vi "RP convert sweep.vi"(6 "Compact":bool, 7 "Desimate result":i32, 11 "FIFO":i32[](array[numeric])) -> (1 "F out":dbl[](array[numeric]), 2 "Y out":dbl[](array[numeric]), 3 "X out":dbl[](array[numeric]))   [LabVIEW 2015]
uses:
  <vilib>/Analysis/2dsp.llb/Decimate (single shot, DBL).vi
  <vilib>/Analysis/NI_AALPro.lvlib
panel:
  in  "Frequency scale":dbl=34.359738368 format="%#_13g"
  in  "Voltage scale":dbl=1e-05
  out "Numeric Control":i32
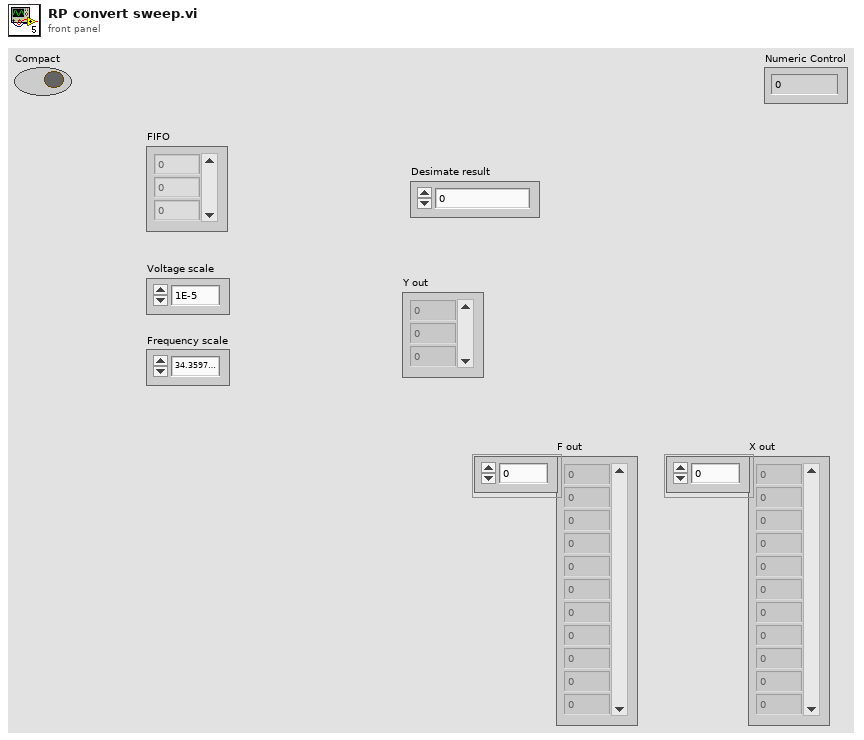
[diagram p1: front panel]
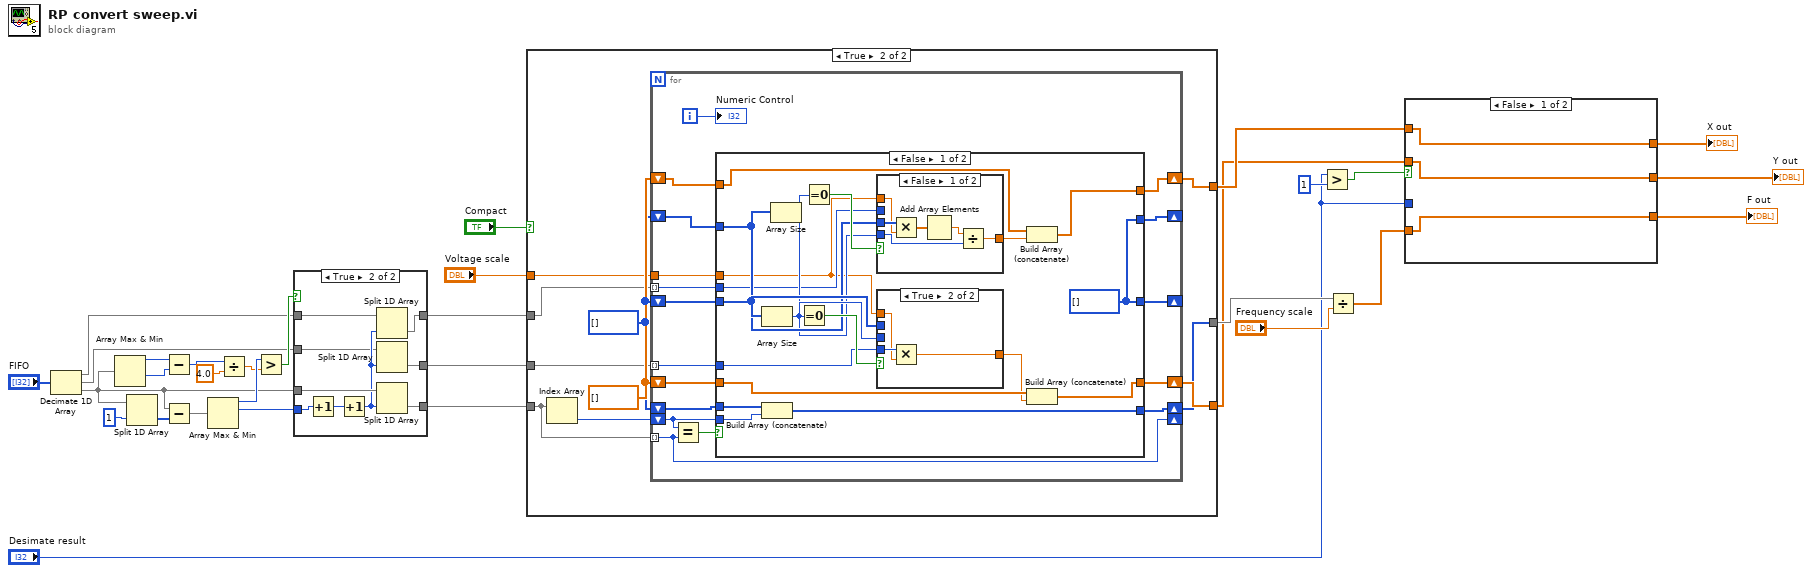
[diagram p0: block diagram]
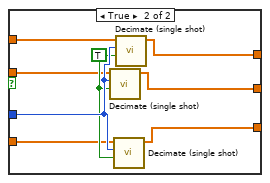
[diagram p2: hidden frame]
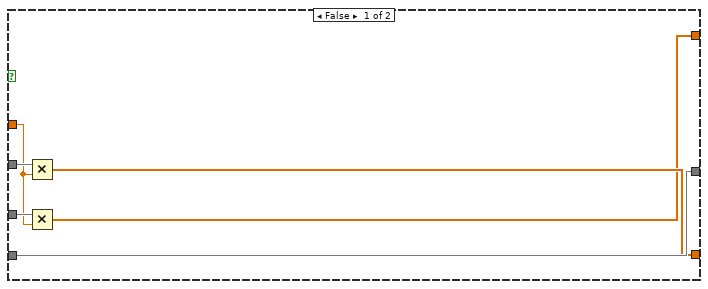
[diagram p3: hidden frame]
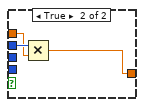
[diagram p4: hidden frame]
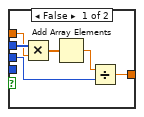
[diagram p5: hidden frame]
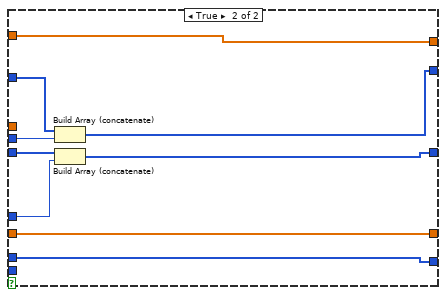
[diagram p6: hidden frame]
diagram:
  n1 = Decimate 1D Array("FIFO") -> (w15:i32[], w13:i32[], w16:i32[])
  n2 = Array Max & Min(array=w16) -> (max value=w28:i32, min value=w27:i32)  [unwired: 2 out]
  n3 = Split 1D Array(array=w16, index=1) -> (second subarray=w30:i32[])  [unwired: 1 out]
  n4 = Subtract(x=w28, y=w27) -> (x-y=w26:i32)
  n5 = Subtract(x=w16, y=w30) -> (x-y=w29:i32[])
  n6 = Array Max & Min(array=w29) -> (max value=w24:i32, max index (indices)=w21:i32)  [unwired: 2 out]
  n7 = Divide(x=w26, y=4.0) -> (x/y=w23:dbl)
  n8 = Greater?(x=w24, y=w23) -> (0:w22:bool)
  n9 = case shown="True" w22 {
    tunnel: w21 -> [_ w43]
    tunnel: w16 -> [w32 w41]
    tunnel: [w32 w40] -> w18
    tunnel: w15 -> [w33 w39]
    tunnel: [w33 w37] -> w20
    tunnel: w13 -> [w34 w36]
    tunnel: [w34 w35] -> w19
    frame False {
    }
    frame True {
      n10 = Increment(x=w43) -> (x+1=w42:i32)
      n11 = Increment(x=w42) -> (x+1=w38:i32)
      n12 = Split 1D Array(array=w39, index=w38) -> (second subarray=w37:i32[])  [unwired: 1 out]
      n13 = Split 1D Array(array=w36, index=w38) -> (second subarray=w35:i32[])  [unwired: 1 out]
      n14 = Split 1D Array(array=w41, index=w38) -> (second subarray=w40:i32[])  [unwired: 1 out]
    }
  }
  n15 = case shown="True" "Compact" {
    tunnel: [w46 w57] -> w6
    tunnel: [w47 w56] -> w5
    tunnel: w20 -> [w48 w55]
    tunnel: w19 -> [w45 w54]
    tunnel: w18 -> [w49 w53]
    tunnel: "Voltage scale" -> [w44 w51]
    tunnel: [w49 w50] -> w12
    frame False {
      n16 = Multiply(x=w48, y=w44) -> (x*y=w47:dbl[])
      n17 = Multiply(x=w45, y=w44) -> (x*y=w46:dbl[])
    }
    frame True {
      w52 = i32[] [] ("Y")
      w58 = dbl[] [] ("Y")
      n18 = Index Array(array=w53) -> (element=w59:i32)  [unwired: 1 in]
      n19 = for {
        tunnel: w53 -> [w62] mode=indexing
        shift-right: [w62] -> _
        shift-left: w59 -> [w64]
        shift-right: [w71] -> _
        shift-left: w52 -> [w73]
        shift-right: [w72] -> _
        shift-left: w52 -> [w76]
        tunnel: w55 -> [w75] mode=indexing
        tunnel: w54 -> [w74] mode=indexing
        shift-right: [w68] -> w57
        shift-left: w58 -> [w69]
        shift-right: [w66] -> w56
        shift-left: w58 -> [w67]
        shift-right: [w63] -> w50
        shift-left: w52 -> [w65]
        tunnel: w51 -> [w60]
        i -> [w61]
        n20 = Equal?(x=w64, y=w62) -> (x = y?=w70:bool)
        n21 = case shown="False" w70 {
          tunnel: w76 -> [w81 w122]
          tunnel: w75 -> [w78 w121]
          tunnel: w74 -> [w83 w120]
          tunnel: w73 -> [w94 w119]
          tunnel: [w95 w118] -> w72
          tunnel: [w95 w117] -> w71
          tunnel: w69 -> [w93 w116]
          tunnel: [w92 w116] -> w68
          tunnel: w67 -> [w91 w115]
          tunnel: [w89 w115] -> w66
          tunnel: w65 -> [w88 w114]
          tunnel: w64 -> [w87 _]
          tunnel: [w86 w114] -> w63
          tunnel: w60 -> [w77 _]
          frame False {
            w95 = i32[] [] ("Y")
            n22 = Array Size(array=w94) -> (size(s)=w85:i32)
            n23 = Build Array (concatenate)(w88, w87) -> (w86:i32[])
            n24 = Array Size(array=w81) -> (size(s)=w79:i32)
            n25 = Equal To 0?(x=w85) -> (x = 0?=w84:bool)
            n26 = Equal To 0?(x=w79) -> (x = 0?=w82:bool)
            n27 = case shown="False" w82 {
              tunnel: w81 -> [w101 _]
              tunnel: [w99 w103] -> w80
              tunnel: w79 -> [w98 _]
              tunnel: w78 -> [_ w104]
              tunnel: w77 -> [w96 w102]
              frame False {
                n28 = Multiply(x=w101, y=w96) -> (x*y=w97:dbl[])
                n29 = Add Array Elements(numeric array=w97) -> (sum=w100:dbl)
                n30 = Divide(x=w100, y=w98) -> (x/y=w99:dbl)
              }
              frame True {
                n31 = Multiply(x=w104, y=w102) -> (x*y=w103:dbl)
              }
            }
            n32 = case shown="True" w84 {
              tunnel: w94 -> [w106 _]
              tunnel: [w109 w112] -> w90
              tunnel: w85 -> [w108 _]
              tunnel: w83 -> [_ w113]
              tunnel: w77 -> [w105 w111]
              frame False {
                n33 = Multiply(x=w106, y=w105) -> (x*y=w107:dbl[])
                n34 = Add Array Elements(numeric array=w107) -> (sum=w110:dbl)
                n35 = Divide(x=w110, y=w108) -> (x/y=w109:dbl)
              }
              frame True {
                n36 = Multiply(x=w113, y=w111) -> (x*y=w112:dbl)
              }
            }
            n37 = Build Array (concatenate)(w93, w80) -> (w92:dbl[])
            n38 = Build Array (concatenate)(w91, w90) -> (w89:dbl[])
          }
          frame True {
            n39 = Build Array (concatenate)(w122, w121) -> (w118:i32[])
            n40 = Build Array (concatenate)(w119, w120) -> (w117:i32[])
          }
        }
        "Numeric Control" <- w61
      }
    }
  }
  n41 = Greater?(x="Desimate result", y=1) -> (0:w8:bool)
  n42 = Divide(x=w12, y="Frequency scale") -> (x/y=w4:dbl[])
  n43 = case shown="False" w8 {
    tunnel: "Desimate result" -> [_ w133]
    tunnel: w6 -> [w125 w131]
    tunnel: w5 -> [w124 w130]
    tunnel: w4 -> [w123 w129]
    tunnel: [w125 w128] -> w3
    tunnel: [w123 w127] -> w2
    tunnel: [w124 w126] -> w1
    frame False {
    }
    frame True {
      w132 = TRUE ("averaging")
      n44 = call-poly <vilib>:"Decimate (single shot).vi"("averaging"=w132, "decimating factor"=w133, "X"=w130) -> ("Decimated Array"=w126:dbl[])  [unwired: 7 in, 1 out]
      n45 = call-poly <vilib>:"Decimate (single shot).vi"("averaging"=w132, "decimating factor"=w133, "X"=w129) -> ("Decimated Array"=w127:dbl[])  [unwired: 7 in, 1 out]
      n46 = call-poly <vilib>:"Decimate (single shot).vi"("averaging"=w132, "decimating factor"=w133, "X"=w131) -> ("Decimated Array"=w128:dbl[])  [unwired: 7 in, 1 out]
    }
  }
  "X out" <- w3
  "Y out" <- w1
  "F out" <- w2
